vi "Read Controls from Config File.vi"(8 "error in (no error)":errorcluster, 10 "Control References":refnum<vi>[](array[refnum]), 11 "Configuration File Reference In":T1) -> (0 "error out":errorcluster, 3 "Configuration File Reference Out":T1)   [LabVIEW 2020]
doc: "Reads the values of an array of controls from a configuration file and writes the values to those controls.\nControl References is an array of the references of the controls to be loaded.\n\nThe section name is the name of the VI that holds the control.\nThe key name is the label of the control."
uses:
  <vilib>/Utility/config.llb/Config Data RefNum.ctl
  <vilib>/Utility/config.llb/NI_LVConfig.lvlib
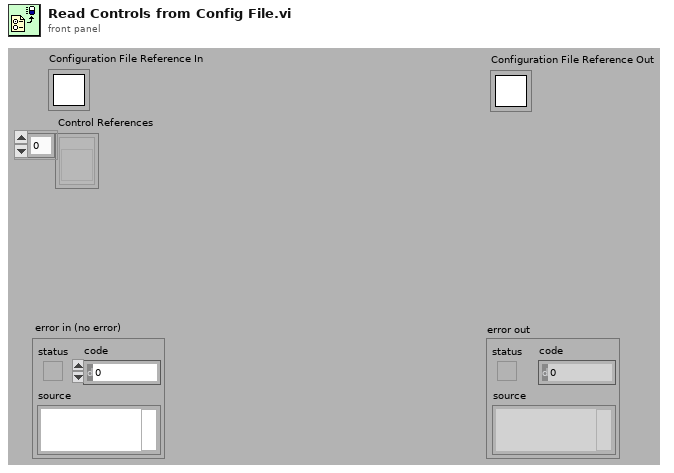
[diagram p1: front panel]
types:
  T1 = typedef "NI_LVConfig.lvlib/Config Data RefNum.ctl" = refnum<k1>
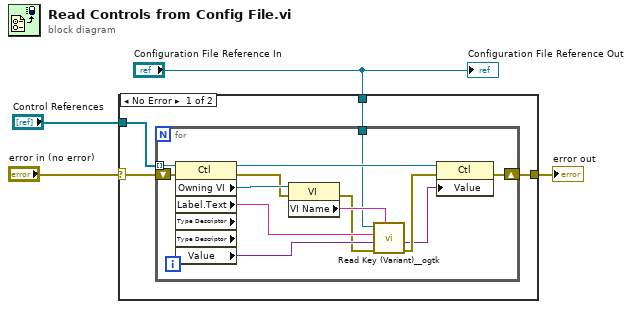
[diagram p0: block diagram]
diagram:
  n1 = case shown="No Error" "error in (no error)" {
    selector: "error in (no error)" -> [w5 w22]
    tunnel: "Control References" -> [w8 _]
    tunnel: [w7 w22] -> w3
    tunnel: "Configuration File Reference In" -> [w6 _]
    frame No Error {
      n2 = for {
        tunnel: w8 -> [w21] mode=indexing
        shift-right: [w17] -> w7
        shift-left: w5 -> [w16]
        tunnel: w6 -> [w14]
        n3 = property class="Ctl" props=["Owning VI", "Label", "Text", "Type Descriptor", "Type Descriptor", "Value"](reference=w21, error in=w16) -> (reference out=w19:refnum<vi>, error out=w18:errorcluster, "Owning VI"=w20:refnum<vi>, "Label.Text"=w13:string, "Value"=w12:variant)  [unwired: 2 out]
        n4 = property class="VI"(reference=w20, error in=w18) -> (error out=w11:errorcluster, "VI Name"=w15:string)  [unwired: 1 out]
        n5 = call <userlib>:"Read Key (Variant)__ogtk.vi"("section"=w15, "error in (no error)"=w11, "type"=w12, "key (optional)"=w13, "refnum"=w14) -> ("error out"=w10:errorcluster, "key-value"=w9:variant)  [unwired: 3 in, 2 out]
        n6 = property class="Ctl"(reference=w19, error in=w10, "Value"=w9) -> (error out=w17:errorcluster)  [unwired: 1 out]
      }
    }
    frame Error {
    }
  }
  "error out" <- w3
  "Configuration File Reference Out" <- "Configuration File Reference In"
